vi "State_Machine.vi"(8 "error in (no error)":errorcluster caption="entrée d'erreur (pas d'erreur)", 11 "Generate_SN en entrée":refnum<class "Find_SN_In_Database.lvclass">) -> (0 "error out":errorcluster caption="sortie d'erreur", 2 "Json_String":string, 3 "Generate_SN en sortie":refnum<class "Find_SN_In_Database.lvclass">)   [LabVIEW 2020, in "Library Test.lvlib" / "Find_SN_In_Database.lvclass"]
uses:
  Find_SN_In_Database.lvclass
  C:/Users/ngarcin/OneDrive - Altyor/Standard TB/Class/Test/Test (Default)/Test (Default).lvclass
  Database/Database Altyor/Database Altyor.lvclass
  JSON API/JSON Value/Set from JSON string.vi
  JSON API/JSON Value/JSON Value.lvclass
  <vilib>/addons/database/_DB Variant To Data/Database Variant To Data.xnode
  Find_SN_In_Database.lvclass/Find_SN_In_Database.ctl
  JSON API/Variant JSON/Variant JSON.lvlib
  JSON API/Get Polymorphic/JSON GetSet.lvlib
panel:
  out "AdditionalInformation":string
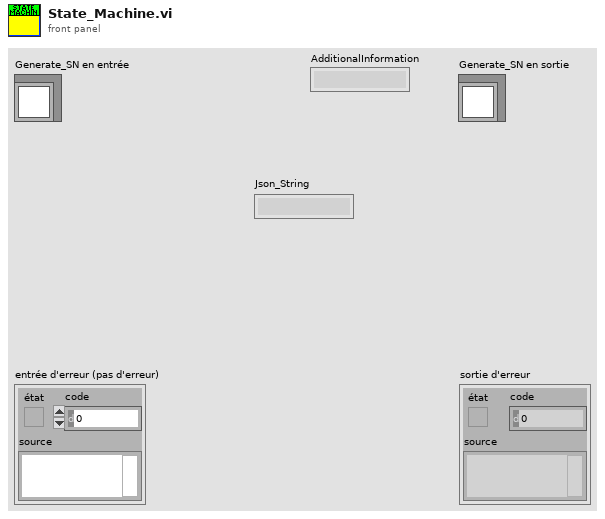
[diagram p1: front panel]
types:
  T1 = cluster{"Connection":string, "Database":string[], "Table":string, "Columm":string, "Value":string}
  T2 = cluster{"Connection":string, "Database":string[], "Table":string, "Line":string}
  T3 = cluster{"idTest":u32, "CreationDate":string, "EndOfProduction":string, "OrderNumber":string, "Batch":string, "ProductName":string, "PartNumber":string, "SerialNumber":string, "Operator":string, "Result":string, "AdditionalInformation":string}[]
  T4 = cluster{"idTest":u32, "CreationDate":string, "EndOfProduction":string, "OrderNumber":string, "Batch":string, "ProductName":string, "PartNumber":string, "SerialNumber":string, "Operator":string, "Result":string, "AdditionalInformation":string}
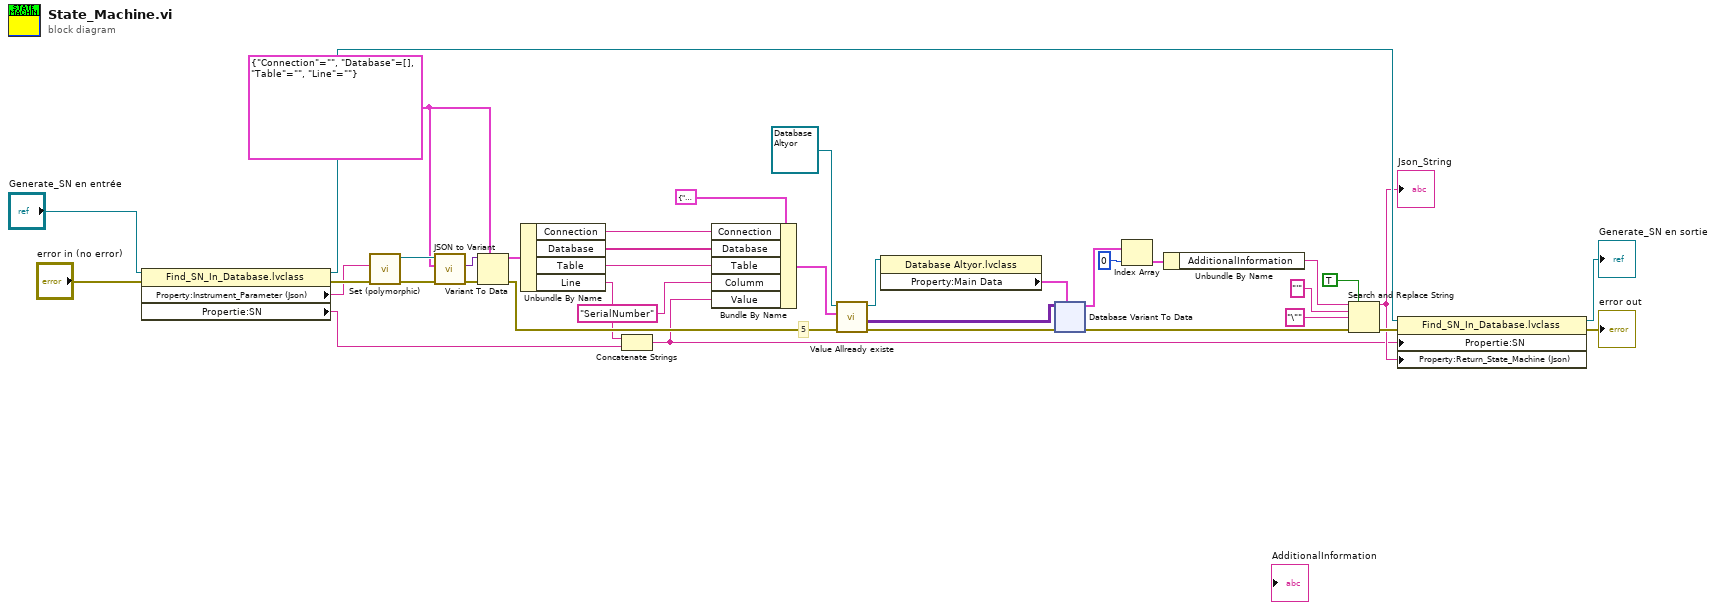
[diagram p0: block diagram]
diagram:
  w29 = T2 {"Connection"="", "Database"=[], "Table"="", "Line"=""} ("Parameter")
  # "5"
  n1 = property class="Find_SN_In_Database.lvclass"(reference="Generate_SN en entrée", error in="error in (no error)") -> (reference out=w27:refnum<class "Find_SN_In_Database.lvclass">, error out=w32:errorcluster, "Property:Instrument_Parameter (Json)"=w30:string, "Propertie:SN"=w2:string)
  n2 = call-poly "Set (polymorphic).vi"("error in (no error)"=w32, "JSON stream"=w30) -> ("error out"=w34:errorcluster, "JSON Value out"=w36:refnum<class "JSON Value.lvclass">)  [unwired: 7 in, 1 out]
  n3 = call "JSON to Variant.vi"("error in (no error)"=w34, "Variant (Data Type)"=w29, "JSON Value"=w36) -> ("error out"=w35:errorcluster, "Variant out"=w33:variant)  [unwired: 7 in]
  n4 = Variant To Data(error in=w35, type=w29, Variant=w33) -> (data=w31:T2, error out=w28:errorcluster)
  n5 = Unbundle By Name(w31) -> ("Connection"=w21:string, "Database"=w20:string[], "Table"=w19:string, "Line"=w15:string)
  n6 = Concatenate Strings(w15, w2) -> (w1:string)
  n7 = Bundle By Name(cluster=T1 {"Connection"="AntennaA", "Database"=["p2313_prod_A_antenna", "p2313_prod_B_antenna"], "Table"="main_table", "Columm"="SerialNumber", "Value"="2313ANT2429B0087"} ("Parameter"), "Connection"=w21, "Database"=w20, "Table"=w19, "Columm"="SerialNumber", "Value"=w1) -> (w18:T1)
  n8 = call-dynamic "Value Allready existe.vi"("error in (no error)"=w28, "Parameter"=w18, "Database Altyor en entrée"=refnum<class "Database Altyor.lvclass"> refnum) -> ("error out"=w11:errorcluster, "Data_Read"=w13:variant[][], "Database Altyor en sortie"=w14:refnum<class "Database Altyor.lvclass">)  [unwired: 5 in, 1 out]
  n9 = property class="Database Altyor.lvclass"(reference=w14) -> ("Property:Main Data"=w12:T3)  [unwired: 1 in, 2 out]
  n10 = xnode "Database Variant To Data"("database variant"=w13, "error in (no error)"=w11, "type"=w12) -> ("data"=w10:T3, "error out"=w3:errorcluster)
  n11 = Index Array(array=w10, index=0 ("indice")) -> (element=w8:T4)
  n12 = Unbundle By Name(w8) -> ("AdditionalInformation"=w7:string)
  n13 = Search and Replace String(replace all?=TRUE ("tout remplacer ? (F)"), input string=w7, search string="'" ("chaîne recherchée"), replace string="\"" ("chaîne de remplacement (\"\")"), error in=w3) -> (result string=w23:string, error out=w26:errorcluster)  [unwired: 3 in, 2 out]
  "Json_String" <- w23
  n14 = property class="Find_SN_In_Database.lvclass"(reference=w27, error in=w26, "Propertie:SN"=w1, "Property:Return_State_Machine (Json)"=w23) -> (reference out=→"Generate_SN en sortie":refnum<class "Find_SN_In_Database.lvclass">, error out=→"error out":errorcluster)
